vi "GOOP4_Base_Create.vi"(8 "error in (no error)":errorcluster, 10 "i":i32, 11 "reference in":refnum<class "GOOP4_Base.lvclass">) -> (0 "error out":errorcluster, 3 "reference out":refnum<class "GOOP4_Base.lvclass">)   [LabVIEW 2012, in "GOOP4_Base.lvclass"]
uses:
  GOOP4_Base.lvclass
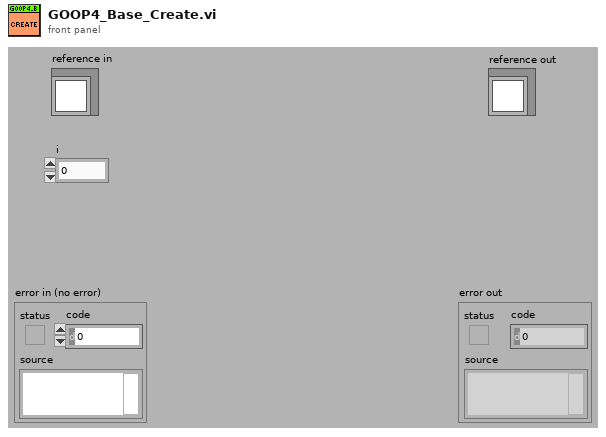
[diagram p1: front panel]
types:
  T1 = typedef "GOOP4_Base.lvclass/ObjectAttributes.ctl" = cluster{"i":i32}
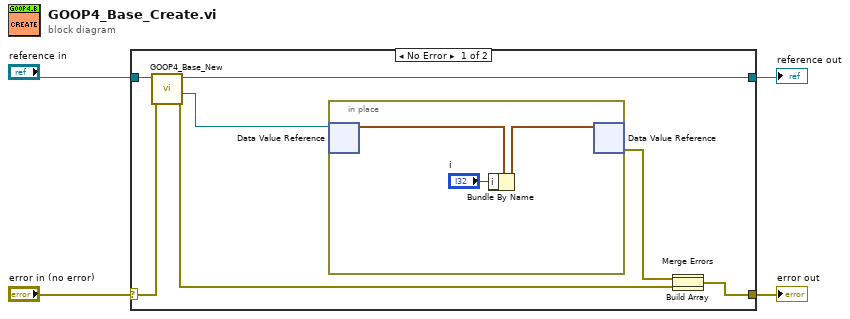
[diagram p0: block diagram]
diagram:
  n1 = case shown="No Error" "error in (no error)" {
    selector: "error in (no error)" -> [w11 w17]
    tunnel: [w8 w17] -> w3
    tunnel: "reference in" -> [w12 w16]
    tunnel: [w10 w16] -> w1
    frame No Error {
      n2 = call "GOOP4_Base_New.vi"("error in (no error)"=w11, "reference in"=w12) -> ("error out"=w7:errorcluster, "DVRRefOut"=w6:refnum<data-value>, "reference out"=w10:refnum<class "GOOP4_Base.lvclass">)  [unwired: 6 in, 1 out]
      n3 = in-place {
        n4 = in-place-dvr #1(w6) -> (w14:T1)  [unwired: 1 out]
        n5 = Bundle By Name(cluster=w14, "i"="i") -> (w15:T1)
        n6 = in-place-dvr #1(w15) -> (w9:errorcluster)  [unwired: 1 out]
      }
      n7 = Build Array(w9, w7) -> (w5:errorcluster[])
      n8 = Merge Errors(w5) -> (w8:errorcluster)
    }
    frame Error {
    }
  }
  "error out" <- w3
  "reference out" <- w1
